vi "Connect to Device.vi"(8 "error in (no error)":errorcluster, 11 "Params":T1={"ID"=0, "SN"="", "Protocol"=enum."SWD", "JTAG_Freq"=enum."9.0 MHz", "SWD_Freq"=enum."4.0 MHz", "Reset_Mode"=enum."UR", "Enable LowPower"=TRUE}) -> (0 "error out":errorcluster, 2 "Connected OK?":bool, 3 "Device ID":string)   [LabVIEW 2015, in "ST-Link.lvlib"]
doc: "根据指定的参数，连接待烧录的芯片，并返回芯片ID和连接状态。\nParams:\n ID: 设备ID，从0~9，根据连接的ST-Link数量自动递增；\n SN：烧录器的SN，可以通过 List ST-Link Infors.vi进行获取，连接时 ID和SN二选一；\n Protocal：选择JTAG或SWD接口协议；\n JTAG_Freq: 设置支持的速率，Protocal为JTAG时需要指定；\n SWD: 设置支持的速率，Protocal为SWD时需要指定；\n Reset_Mode: 指定复位模式，UR或HOTPLUG；\n Enable LowPower: 是否使能低功耗模式；\n\n[Device ID]: 返回连接上的芯片ID；\n[Connected OK?]: 返回连接状态，OK or NG；"
uses:
  ST-Link.lvlib
panel:
  out "standard output":string
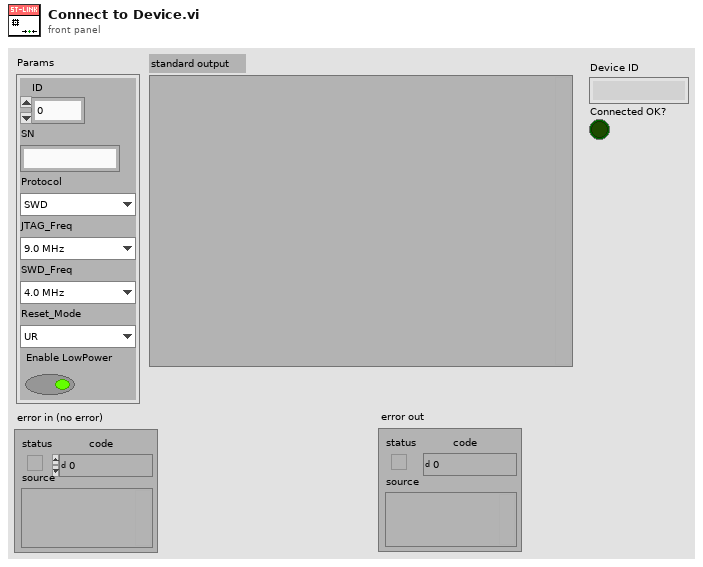
[diagram p1: front panel]
types:
  T1 = cluster{"ID":u8, "SN":string, "Protocol":enum16{"JTAG", "SWD"}, "JTAG_Freq":enum16{"9.0 MHz", "140 KHz", "281 KHz", "562 KHz", "1125 KHz", "2250 KHz", "4500 KHz"}, "SWD_Freq":enum16{"4.0 MHz", "005 KHz", "015 KHz", "025 KHz", "050 KHz", "100 KHz", "125 KHz", "240 KHz", "480 KHz", "0.9 MHz", "1.8 MHz"}, "Reset_Mode":enum16{"UR", "HOTPLUG"}, "Enable LowPower":bool}
  T2 = enum16{"9.0 MHz", "140 KHz", "281 KHz", "562 KHz", "1125 KHz", "2250 KHz", "4500 KHz"}
  T3 = enum16{"4.0 MHz", "005 KHz", "015 KHz", "025 KHz", "050 KHz", "100 KHz", "125 KHz", "240 KHz", "480 KHz", "0.9 MHz", "1.8 MHz"}
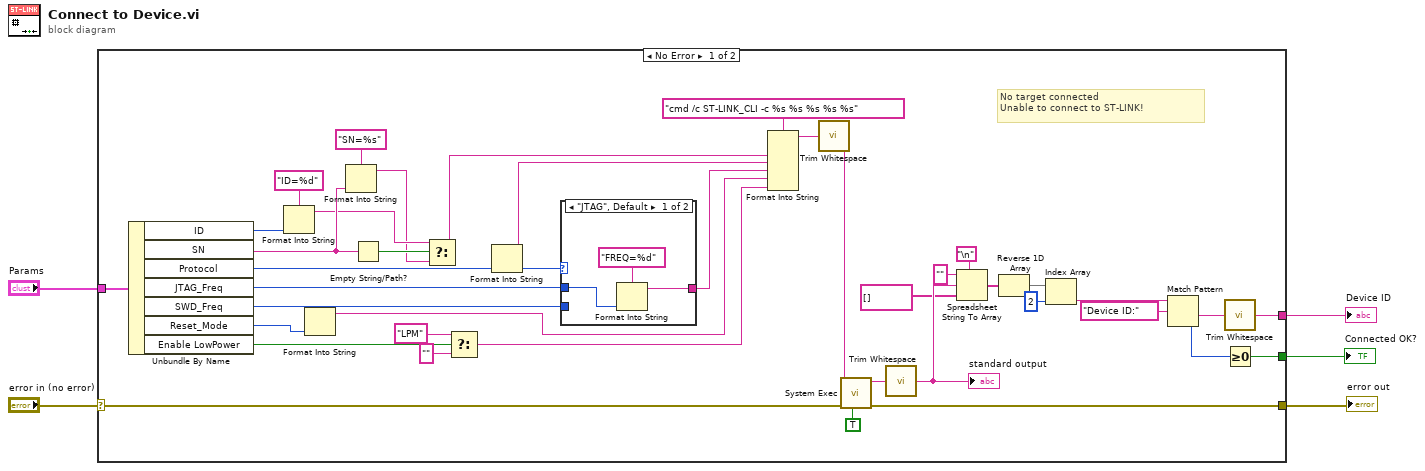
[diagram p0: block diagram]
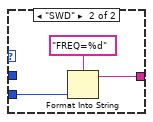
[diagram p2: hidden frame]
diagram:
  n1 = case shown="No Error" "error in (no error)" {
    selector: "error in (no error)" -> [w44 w52]
    tunnel: [w43 w52] -> w4
    tunnel: "Params" -> [w41 _]
    tunnel: [w8 _] -> w2
    tunnel: [w6 _] -> w1
    frame No Error {
      # "No target connected\nUnable to connect to ST-LINK!"
      n2 = Unbundle By Name(w41) -> ("ID"=w38:u8, "SN"=w36:string, "Protocol"=w33:enum16{"JTAG", "SWD"}, "JTAG_Freq"=w32:T2, "SWD_Freq"=w31:T3, "Reset_Mode"=w30:enum16{"UR", "HOTPLUG"}, "Enable LowPower"=w29:bool)
      n3 = Format Into String(format string="ID=%d", w38) -> (resulting string=w35:string)  [unwired: 2 in, 1 out]
      n4 = Format Into String(w30) -> (resulting string=w22:string)  [unwired: 3 in, 1 out]
      n5 = Format Into String(format string="SN=%s", w36) -> (resulting string=w34:string)  [unwired: 2 in, 1 out]
      n6 = Empty String/Path?(string/path=w36) -> (empty?=w40:bool)
      n7 = Select(t=w35, s=w40, f=w34) -> (s? t:f=w25:string)
      n8 = Select(t="LPM", s=w29, f="") -> (s? t:f=w21:string)
      n9 = Format Into String(w33) -> (resulting string=w24:string)  [unwired: 3 in, 1 out]
      n10 = case shown="\"JTAG\", Default" w33 {
        tunnel: w32 -> [w46 _]
        tunnel: w31 -> [_ w50]
        tunnel: [w47 w49] -> w23
        frame "JTAG", Default {
          n11 = Format Into String(format string="FREQ=%d", w46) -> (resulting string=w47:string)  [unwired: 2 in, 1 out]
        }
        frame "SWD" {
          n12 = Format Into String(format string="FREQ=%d", w50) -> (resulting string=w49:string)  [unwired: 2 in, 1 out]
        }
      }
      n13 = Format Into String(format string="cmd /c ST-LINK_CLI -c %s %s %s %s %s" ("command line"), w25, w24, w23, w22, w21) -> (resulting string=w20:string)  [unwired: 2 in, 1 out]
      n14 = call <vilib>:"Trim Whitespace.vi"("string"=w20) -> ("trimmed string"=w19:string)  [unwired: 1 in]
      n15 = call <vilib>:"System Exec.vi"("run minimized? (F)"=TRUE, "error in (no error)"=w44, "command line"=w19) -> ("error out"=w43:errorcluster, "standard output"=w42:string)  [unwired: 5 in, 2 out]
      n16 = call <vilib>:"Trim Whitespace.vi"("string"=w42) -> ("trimmed string"=w18:string)  [unwired: 1 in]
      "standard output" <- w18
      n17 = Spreadsheet String To Array(delimiter (Tab)="\n", format string="", spreadsheet string=w18, array type (2D Dbl)=string[] []) -> (array=w14:string[])
      n18 = Reverse 1D Array(array=w14) -> (reversed array=w13:string[])
      n19 = Index Array(array=w13, index=2) -> (element=w11:string)
      n20 = Match Pattern(string=w11, regular expression="Device ID:") -> (after substring=w9:string, offset past match=w7:i32)  [unwired: 1 in, 2 out]
      n21 = call <vilib>:"Trim Whitespace.vi"("string"=w9) -> ("trimmed string"=w8:string)  [unwired: 1 in]
      n22 = Greater Or Equal To 0?(x=w7) -> (x >= 0?=w6:bool)
    }
    frame Error {
    }
  }
  "error out" <- w4
  "Device ID" <- w2
  "Connected OK?" <- w1
